vi "Create Transfer Sections.vi"(7 "GUID (Default Section)":string="03D3BB89-1485-13A6-56005DE6430FF8B7", 8 "error in (no error)":errorcluster, 10 "Transfer Configurations":refnum<class "Transfer Configuration.lvclass">[](array[class]), 11 "Item Ref in":T1 format="%.0x") -> (0 "error out":errorcluster, 2 "Transfer Section refs":T1[](array[typedef]) format="%.0x", 3 "Item Ref out":T1 format="%.0x")   [LabVIEW 2019, in "DSF System Explorer.lvlib"]
uses:
  DSF System Explorer.lvlib
  <vilib>/NI VeriStand/Custom Device API/Custom Device API.lvlib
  <vilib>/NI VeriStand/Custom Device API/Custom Device Item Ref.ctl
  DSF Core.lvlibp/Classes/Configuration/Core/Transfer/Transfer Configuration.lvclass
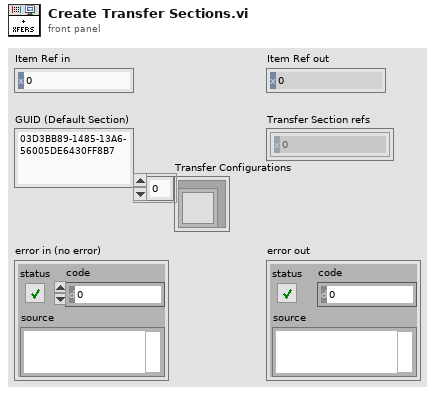
[diagram p1: front panel]
types:
  T1 = typedef "Custom Device API.lvlib/Custom Device Item Ref.ctl" = u64
  T2 = typedef "DSF Core.lvlibp/Transfer Configuration.lvclass/Core Transfer Configuration.ctl" = cluster{"name":string}
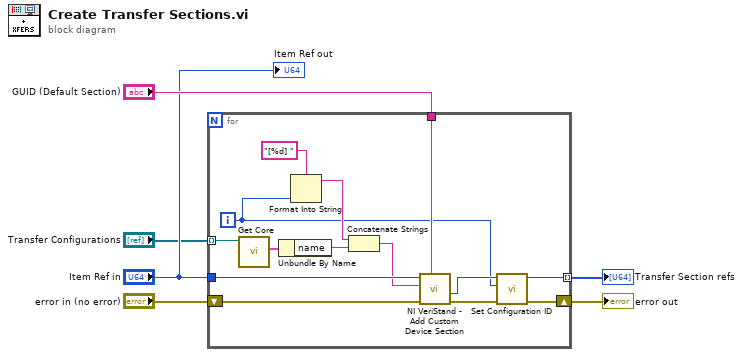
[diagram p0: block diagram]
diagram:
  n1 = for {
    tunnel: "Transfer Configurations" -> [w9] mode=indexing
    tunnel: "Item Ref in" -> [w20]
    shift-right: [w13] -> w6
    shift-left: "error in (no error)" -> [w19]
    tunnel: [w12] -> w5 mode=indexing
    tunnel: "GUID (Default Section)" -> [w11]
    i -> [w10]
    n2 = call "Get Core.vi"("Transfer Configuration in"=w9) -> ("core"=w8:T2)  [unwired: 8 in, 2 out]
    n3 = Unbundle By Name(w8) -> ("name"=w7:string)
    n4 = Format Into String(format string="[%d] ", w10) -> (resulting string=w17:string)  [unwired: 2 in, 1 out]
    n5 = Concatenate Strings(w17, w7) -> (w16:string)
    n6 = call <vilib>:"NI VeriStand - Add Custom Device Section.vi"("GUID (Default Section)"=w11, "error in (no error)"=w19, "Section Name"=w16, "Parent Ref in"=w20) -> ("error out"=w18:errorcluster, "Section Ptr"=w14:T1)  [unwired: 4 in, 2 out]
    n7 = call "Set Configuration ID.vi"("error in (no error)"=w18, "Configuration ID"=w10, "Item Ref in"=w14) -> ("error out"=w13:errorcluster, "Item Ref out"=w12:T1)  [unwired: 7 in]
  }
  "error out" <- w6
  "Transfer Section refs" <- w5
  "Item Ref out" <- "Item Ref in"
